vi "DFD MRate Filtering (Array NChan).vi"(6 "zero phase? (T)":bool=TRUE, 7 "init? (F)":bool, 8 "error in (no error)":errorcluster, 10 "multirate filter":T1={"mMRate_Structure"=enum."IIR", "mMRate_Mode"=0, "mMRate_Factor"=-1, "mMRate_FIRParams"={"mMRate_FIR_H"=[], "mMRate_FIR_IsNyquist?"=FALSE, "mMRate_FIR_IsSymmetric?"=FALSE}, "mMRate_CICParams"={"mMRate_CIC_#Stage"=0, "mMRate_CIC_Lag"=0, "mMRate_CIC_Type"=enum."Lowpass"}, "mMRate_Order"=0, "mMRate_Version"="2.0", "mMRate_Comments"="", "mMRate_RationalFactor"={"mMRate_L"=-1, "mMRate_M"=-1}, "mMRate_Fs"=1.0, "mMRate_Quantized?"=FALSE, "mMRate_QFilterGain"=1.0, "mMRate_CoefWl"=16, "mMRate_Scaling"={"mMRate_ScaleByPowerOf2?"=FALSE, "mMRate_ScaleType"=enum."No Norm"}, "mMRate_InputWl"=16, "mMRate_OutputWl"=16, "mMRate_OutputMode"=enum."Truncation", "mMRate_MultMode"=enum."Truncated", "mMRate_BitPruning"=FALSE, "mMRate_GainWl"=16, "mMRate_OutputFwl"=0, "mMRate_SumIwl"=0, "mMRate_InputIwl "=16, "mMRate_SumWl"=32, "mMRate_CoefIwl"=0} {"mMRate_SumWl" min=1 max=32 step=1; "mMRate_InputIwl" min=1 max=32 step=1; "mMRate_GainWl" min=1 max=32 step=1; "mMRate_OutputWl" min=1 max=32 step=1; "mMRate_InputWl" min=1 max=32 step=1; "mMRate_CoefWl" min=1 max=32 step=1; "mMRate_Mode" items=["Default"=-1, "No Rate Change"=0, "Interpolation"=1, "Decimation"=2, "Interpolated"=3, "Rational"=4]}, 11 "signal in":dbl[][](array[numeric])) -> (0 "error out":errorcluster, 3 "signal out":dbl[][](array[numeric]))   [LabVIEW 2017, in "NI_DigFilterLicensed.lvlib"]
doc: "Filters a signal continuously with a multirate filter. Wire data to the <B>signal in</B> input to determine the polymorphic instance to use or manually select the instance."
uses:
  <vilib>/addons/Digital Filter Design/NI_DigFilterLicensed.lvlib
  <vilib>/addons/Digital Filter Design/_Objects.llb/DFD Multirate Filter Obj.ctl
  <vilib>/addons/Digital Filter Design/_Objects.llb/DFD Multirate Mode.ctl
  <vilib>/addons/Digital Filter Design/_Objects.llb/DFD Coef Norm Type.ctl
  <vilib>/addons/Digital Filter Design/_Objects.llb/DFD Round-off Mode.ctl
  <vilib>/addons/Digital Filter Design/_Objects.llb/DFD FXP MRate Multiply Mode.ctl
  <vilib>/addons/Digital Filter Design/NI_DigFilter_Process.lvlib
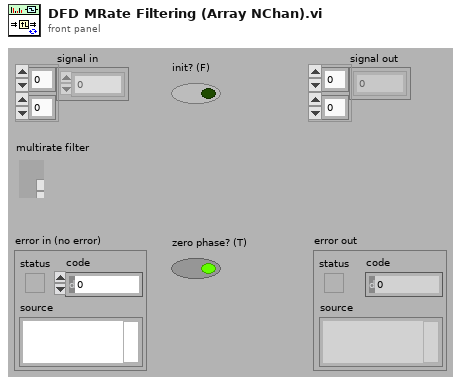
[diagram p1: front panel]
types:
  T1 = typedef "NI_DigFilterLicensed.lvlib/DFD Multirate Filter Obj.ctl" = cluster{"mMRate_Structure":enum16{"CIC", "FIR", "IIR", "Lattice"}, "mMRate_Mode":T2, "mMRate_Factor":i32, "mMRate_FIRParams":cluster{"mMRate_FIR_H":dbl[], "mMRate_FIR_IsNyquist?":bool, "mMRate_FIR_IsSymmetric?":bool}, "mMRate_CICParams":cluster{"mMRate_CIC_#Stage":i32, "mMRate_CIC_Lag":i32, "mMRate_CIC_Type":enum16{"Lowpass", "Highpass"}}, "mMRate_Order":i32, "mMRate_Version":string, "mMRate_Comments":string, "mMRate_RationalFactor":cluster{"mMRate_L":i32, "mMRate_M":i32}, "mMRate_Fs":dbl, "mMRate_Quantized?":bool, "mMRate_QFilterGain":dbl, "mMRate_CoefWl":i16, "mMRate_Scaling":cluster{"mMRate_ScaleByPowerOf2?":bool, "mMRate_ScaleType":T3}, "mMRate_InputWl":i16, "mMRate_OutputWl":i16, "mMRate_OutputMode":T4, "mMRate_MultMode":T5, "mMRate_BitPruning":bool, "mMRate_GainWl":i16, "mMRate_OutputFwl":i16, "mMRate_SumIwl":i16, "mMRate_InputIwl ":i16, "mMRate_SumWl":i16, "mMRate_CoefIwl":i16}
  T2 = typedef "NI_DigFilterLicensed.lvlib/DFD Multirate Mode.ctl" = i16
  T3 = typedef "NI_DigFilterLicensed.lvlib/DFD Coef Norm Type.ctl" = enum16{"No Norm", "Time Domain 1-Norm", "Time Domain 2-Norm", "Time Domain Inf-Norm"}
  T4 = typedef "NI_DigFilterLicensed.lvlib/DFD Round-off Mode.ctl" = enum16{"Nearest", "Truncation"}
  T5 = typedef "NI_DigFilterLicensed.lvlib/DFD FXP MRate Multiply Mode.ctl" = enum16{"Truncated", "Full"}
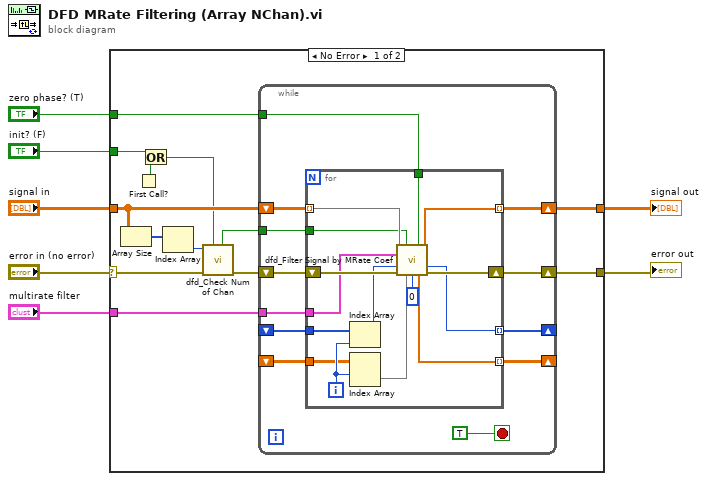
[diagram p0: block diagram]
diagram:
  n1 = case shown="No Error" "error in (no error)" {
    selector: "error in (no error)" -> [w11 w48]
    tunnel: [w19 w48] -> w5
    tunnel: "multirate filter" -> [w20 _]
    tunnel: "signal in" -> [w15 _]
    tunnel: "zero phase? (T)" -> [w18 _]
    tunnel: "init? (F)" -> [w16 _]
    tunnel: [w9 _] -> w1
    frame No Error {
      n2 = Array Size(array=w15) -> (size(s)=w14:i32[])
      n3 = First Call?() -> (First Call?: T/F=w17:bool)
      n4 = Or(x=w16, y=w17) -> (x .or. y?=w12:bool)
      n5 = Index Array(array=w14) -> (element=w13:i32)  [unwired: 1 in]
      n6 = call <vilib>:"dfd_Check Num of Chan.vi"("init in"=w12, "error in (no error)"=w11, "#ch in"=w13) -> ("error out"=w10:errorcluster, "init out"=w8:bool)  [unwired: 7 out]
      n7 = while {
        tunnel: w20 -> [w32]
        shift-right: [w24] -> _
        shift-left: _ -> [w25]
        tunnel: w18 -> [w21]
        shift-right: [w27] -> _
        shift-left: _ -> [w26]
        shift-right: [w28] -> w19
        shift-left: w10 -> [w30]
        tunnel: w8 -> [w22]
        shift-right: [w23] -> w9
        shift-left: w15 -> [w29]
        stop <- TRUE stop-if-true
        n8 = for {
          tunnel: w32 -> [w44]
          tunnel: w29 -> [w47] mode=indexing
          shift-right: [w45] -> w28
          shift-left: w30 -> [w46]
          tunnel: [w43] -> w27 mode=indexing
          tunnel: w26 -> [w42]
          tunnel: w25 -> [w38]
          tunnel: [w37] -> w24 mode=indexing
          tunnel: [w35] -> w23 mode=indexing
          tunnel: w22 -> [w34]
          tunnel: w21 -> [w33]
          i -> [w40]
          n9 = Index Array(array=w42, index=w40) -> (element=w41:i32)
          n10 = Index Array(array=w38, index (row)=w40) -> (element=w39:dbl[])  [unwired: 1 in]
          n11 = call <vilib>:"dfd_Filter Signal by MRate Coef.vi"("signal in"=w47, "initH?"=w34, "zeroPhaseH?"=w33, "multirate filter"=w44, "skipPoint In"=w41, "error in (no error)"=w46, "state in"=w39, "outputPhase"=0) -> ("signal out"=w35:dbl[], "skipPoint Out"=w43:i32, "state out"=w37:dbl[], "error out"=w45:errorcluster)  [unwired: 4 out]
        }
      }
    }
    frame Error {
    }
  }
  "error out" <- w5
  "signal out" <- w1
